vi "gaussian correlation time old.vi"() -> ()   [LabVIEW 2014]
uses:
  <vilib>/userdefined/High Color/IMAQdx.ctl
  <vilib>/Utility/file.llb/Write To Spreadsheet File (DBL).vi
  <vilib>/Utility/file.llb/Read From Spreadsheet File (string).vi
  <vilib>/vision/driver/NI_Vision_Acquisition_Software.lvlib
panel:
  in  "Transfer and Run Date Folder After Experiment":bool
  in  "SSH user name":string
  in  "SSH password":string
  in  "Tags":string
  in  "Wait before recording (s)":dbl
  in  "Correlation Time (s)":dbl
  in  "Start Recording":bool
  in  "Max Power (uW/mm^2)":dbl
  in  "Min Power (uW/mm^2)":dbl
  in  "Frames":i32
  in  "Sigma (uW/mm^2)":dbl
  in  "Offset Power (uW/mm^2)":dbl
  out "Error":string
  out "Save Directory":path
  out "Buffer Number Out":u32
  out "Image":T1(plugin-control)
  in  "stop":bool
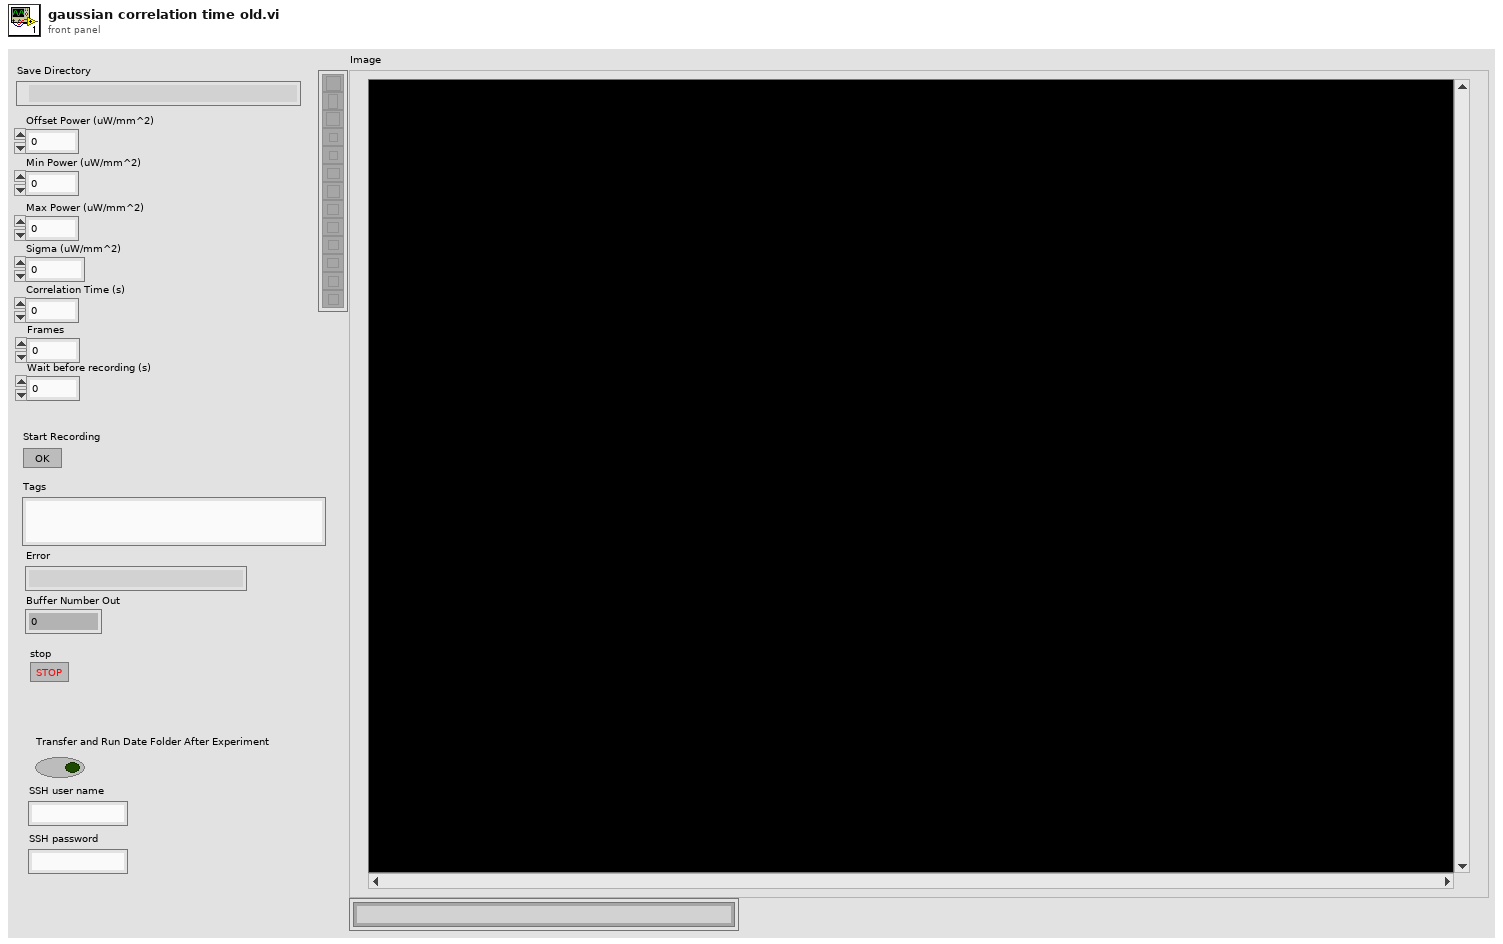
[diagram p1: front panel]
types:
  T1 = typedef "IMAQ Image.ctl" = refnum<image>
  T2 = typedef "IMAQdx.ctl" = refnum<k21>
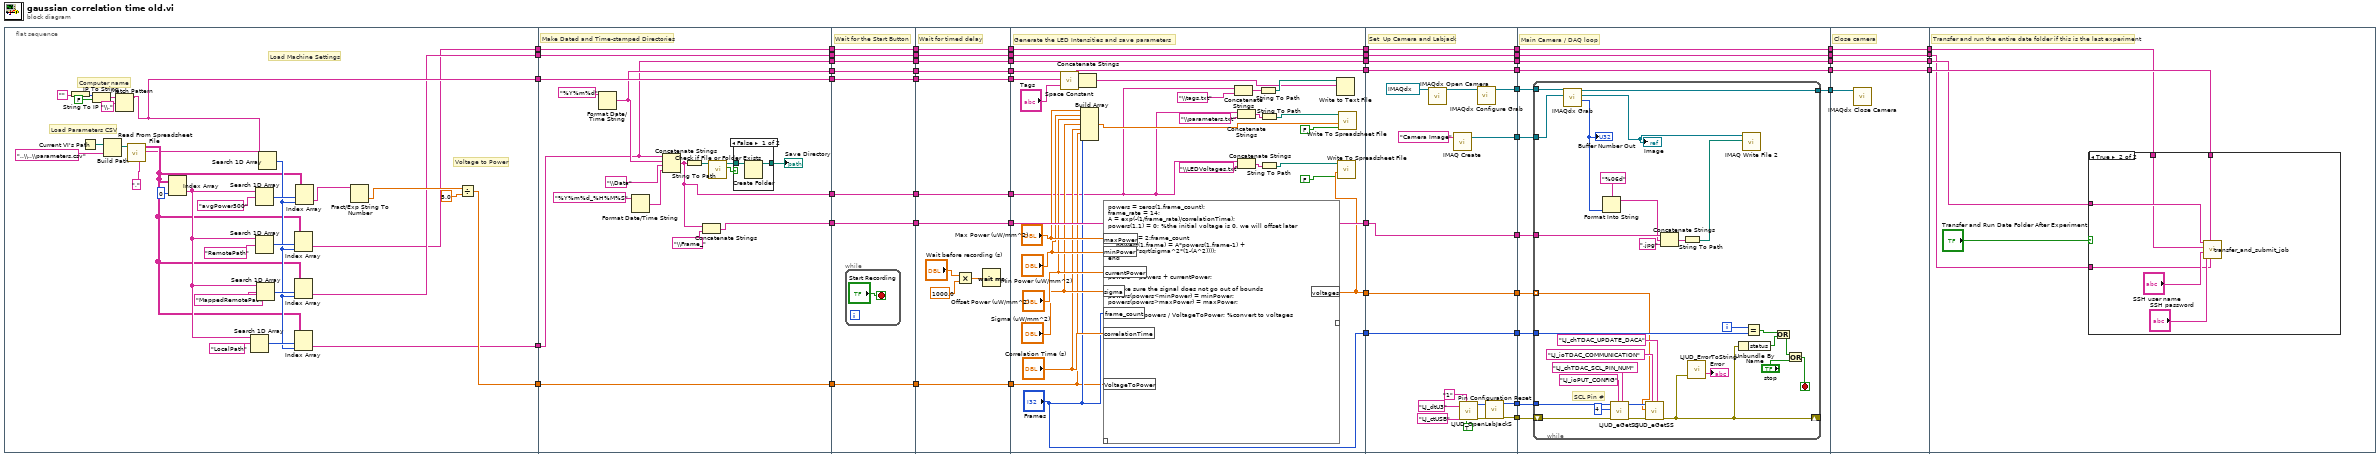
[diagram p0: block diagram]
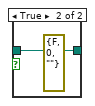
[diagram p2: hidden frame]
diagram:
  n1 = flat-sequence {
    tunnel: [w78] -> w36
    tunnel: [w77] -> w32
    tunnel: [w64] -> w17
    tunnel: [w63] -> w16
    tunnel: [w62] -> w15
    tunnel: [w95] -> w45
    tunnel: [w93] -> w44
    tunnel: [w92] -> w37
    tunnel: w36 -> [w92]
    tunnel: [w91] -> w33
    tunnel: w32 -> [w91]
    tunnel: [w90] -> w29
    tunnel: [w89] -> w24
    tunnel: w17 -> [w89]
    tunnel: w16 -> [w87]
    tunnel: w15 -> [w88]
    tunnel: [w88] -> w8
    tunnel: [w87] -> w1
    tunnel: w45 -> [w114]
    tunnel: [w114] -> w43
    tunnel: w44 -> [w113]
    tunnel: [w113] -> w41
    tunnel: [w112] -> w38
    tunnel: w37 -> [w112]
    tunnel: [w111] -> w34
    tunnel: w33 -> [w111]
    tunnel: [w110] -> w30
    tunnel: w29 -> [w110]
    tunnel: w24 -> [w109]
    tunnel: [w109] -> w18
    tunnel: [w108] -> w9
    tunnel: w8 -> [w108]
    tunnel: [w107] -> w2
    tunnel: w1 -> [w107]
    tunnel: w43 -> [w126]
    tunnel: [w126] -> w42
    tunnel: w41 -> [w125]
    tunnel: [w125] -> w40
    tunnel: [w121] -> w39
    tunnel: w38 -> [w121]
    tunnel: [w120] -> w35
    tunnel: w34 -> [w120]
    tunnel: [w119] -> w31
    tunnel: w30 -> [w119]
    tunnel: [w118] -> w19
    tunnel: w18 -> [w118]
    tunnel: [w117] -> w10
    tunnel: w9 -> [w117]
    tunnel: [w116] -> w3
    tunnel: w2 -> [w116]
    tunnel: w42 -> [w154]
    tunnel: [w154] -> w50
    tunnel: [w152] -> w48
    tunnel: ["Frames"] -> w47
    tunnel: w40 -> [w138]
    tunnel: w39 -> [w139]
    tunnel: w35 -> [w134]
    tunnel: w31 -> [w130]
    tunnel: [w130] -> w25
    tunnel: [w129] -> w20
    tunnel: w19 -> [w129]
    tunnel: [w128] -> w11
    tunnel: w10 -> [w128]
    tunnel: [w127] -> w4
    tunnel: w3 -> [w127]
    tunnel: w50 -> [w171]
    tunnel: [w173] -> w56
    tunnel: [w172] -> w55
    tunnel: [w171] -> w54
    tunnel: [w163] -> w52
    tunnel: [w162] -> w51
    tunnel: [w167] -> w49
    tunnel: w48 -> [w167]
    tunnel: w47 -> [w166]
    tunnel: [w166] -> w46
    tunnel: [w160] -> w26
    tunnel: w25 -> [w160]
    tunnel: [w159] -> w21
    tunnel: w20 -> [w159]
    tunnel: [w158] -> w12
    tunnel: w11 -> [w158]
    tunnel: [w157] -> w5
    tunnel: w4 -> [w157]
    tunnel: w56 -> [w188]
    tunnel: w55 -> [w187]
    tunnel: w54 -> [w186]
    tunnel: [w185] -> w53
    tunnel: w52 -> [w184]
    tunnel: w51 -> [w183]
    tunnel: w49 -> [w182]
    tunnel: w46 -> [w181]
    tunnel: [w180] -> w27
    tunnel: w26 -> [w180]
    tunnel: [w179] -> w22
    tunnel: w21 -> [w179]
    tunnel: [w178] -> w13
    tunnel: w12 -> [w178]
    tunnel: [w177] -> w6
    tunnel: w5 -> [w177]
    tunnel: w53 -> [w223]
    tunnel: [w222] -> w28
    tunnel: w27 -> [w222]
    tunnel: [w221] -> w23
    tunnel: w22 -> [w221]
    tunnel: [w220] -> w14
    tunnel: w13 -> [w220]
    tunnel: [w219] -> w7
    tunnel: w6 -> [w219]
    tunnel: w28 -> [w227]
    tunnel: w23 -> [w226]
    tunnel: w14 -> [w225]
    tunnel: w7 -> [w224]
    frame #0 {
      # "Voltage to Power"
      # "Load Parameters CSV"
      # "Computer name"
      # "Load Machine Settings"
      n2 = String To IP(1:"") -> (0:w86:u32)
      n3 = Current VI's Path() -> (path=w81:path)
      n4 = IP To String(1:FALSE, 2:w86) -> (0:w83:string)
      n5 = Build Path(base path=w81, name or relative path="..\\..\\parameters.csv") -> (appended path=w60:path)
      n6 = Match Pattern(string=w83, regular expression="\\.") -> (before substring=w77:string)  [unwired: 1 in, 3 out]
      n7 = call-poly <vilib>:"Read From Spreadsheet File.vi"("delimiter (\\t)"=",", "file path (dialog if empty)"=w60) -> ("first row"=w58:string[], "all rows"=w59:string[][])  [unwired: 5 in, 3 out]
      n8 = Index Array(array=w59, index (col)=0) -> (element=w61:string[])  [unwired: 1 in]
      n9 = Search 1D Array(1D array=w61, element="LocalPath") -> (index of element=w66:i32)  [unwired: 1 in]
      n10 = Search 1D Array(1D array=w61, element="RemotePath") -> (index of element=w71:i32)  [unwired: 1 in]
      n11 = Search 1D Array(1D array=w61, element="avgPower500") -> (index of element=w72:i32)  [unwired: 1 in]
      n12 = Search 1D Array(1D array=w61, element="MappedRemotePath") -> (index of element=w70:i32)  [unwired: 1 in]
      n13 = Search 1D Array(1D array=w58, element=w77) -> (index of element=w65:i32)  [unwired: 1 in]
      n14 = Index Array(array=w59, index (row)=w71, index (col)=w65) -> (element=w62:string)
      n15 = Index Array(array=w59, index (row)=w70, index (col)=w65) -> (element=w63:string)
      n16 = Index Array(array=w59, index (row)=w66, index (col)=w65) -> (element=w64:string)
      n17 = Index Array(array=w59, index (row)=w72, index (col)=w65) -> (element=w69:string)
      n18 = Fract/Exp String To Number(string=w69) -> (number=w68:dbl)  [unwired: 3 in, 1 out]
      n19 = Divide(x=w68, y=5.0) -> (x/y=w78:dbl)
    }
    frame #1 {
      # "Make Dated and Time-stamped Directories"
      n20 = Format Date/Time String(time format string (%c)="%Y%m%d") -> (date/time string=w90:string)  [unwired: 2 in]
      n21 = Format Date/Time String(time format string (%c)="%Y%m%d_%H%M%S") -> (date/time string=w98:string)  [unwired: 2 in]
      n22 = Concatenate Strings(w89, w90, "\\Data", w98) -> (w93:string)
      n23 = String To Path(string=w93) -> (path=w97:path)
      n24 = Concatenate Strings(w93, "\\Frame_") -> (w95:string)
      n25 = call <vilib>:"Check if File or Folder Exists.vi"("path"=w97) -> ("file or folder exists?"=w102:bool, "dup path"=w101:path)  [unwired: 8 in, 1 out]
      n26 = case shown="False" w102 {
        tunnel: [w104 w106] -> w96
        tunnel: w101 -> [w105 w106]
        frame False {
          n27 = Create Folder(path (use dialog)=w105) -> (created path=w104:path)  [unwired: 2 in, 2 out]
        }
        frame True {
          (unwired) errorcluster {"status"=FALSE, "code"=0, "source"=""} ("error out")
        }
      }
      "Save Directory" <- w96
    }
    frame #2 {
      # "Wait for the Start Button"
      n28 = while {
        stop <- "Start Recording" stop-if-true
      }
    }
    frame #3 {
      # "Wait for timed delay"
      n29 = Multiply(x="Wait before recording (s)", y=1000.0) -> (x*y=w123:dbl)
      n30 = Wait (ms)(milliseconds to wait=w123) -> ()  [unwired: 1 out]
    }
    frame #4 {
      # "Generate the LED Intensities and save parameters"
      n31 = call <vilib>:"Space Constant.vi"() -> ("String"=w132:string)
      n32 = Concatenate Strings(w134, w132, "Tags") -> (w131:string)
      n33 = Build Array("Max Power (uW/mm^2)", "Min Power (uW/mm^2)", "Offset Power (uW/mm^2)", "Sigma (uW/mm^2)", "Correlation Time (s)", w139, "Frames") -> (w142:dbl[])
      n34 = script code="powers = zeros(1,frame_count);\nframe_rate = 14;\nA = exp(-(1/frame_rate)/correlationTime);\npowers(1,1) = 0; %the initial voltage is 0, we will offset later\n\nfor frame = 2:frame_count\n    powers(1,frame) = A*powers(1,frame-1) + (randn(1)*sqrt(sigma^2*(1-(A^2))));\nend\n\n%offset\npowers = powers + currentPower;\n\n%make sure the signal does not go out of bounds\npowers(powers<minPower) = minPower;\npowers(powers>maxPower) = maxPower;\n\nvoltages = powers / VoltageToPower; %convert to voltages"("currentPower"="Offset Power (uW/mm^2)", "frame_count"="Frames", "sigma"="Sigma (uW/mm^2)", "minPower"="Min Power (uW/mm^2)", "maxPower"="Max Power (uW/mm^2)", "correlationTime"="Correlation Time (s)", "VoltageToPower"=w139) -> ("voltages"=w152:dbl[])  [unwired: 1 in, 1 out]
      n35 = Concatenate Strings(w138, "\\tags.txt") -> (w136:string)
      n36 = Concatenate Strings(w138, "\\LEDVoltages.txt") -> (w156:string)
      n37 = Concatenate Strings(w138, "\\parameters.txt") -> (w146:string)
      n38 = String To Path(string=w136) -> (path=w135:path)
      n39 = String To Path(string=w156) -> (path=w155:path)
      n40 = String To Path(string=w146) -> (path=w145:path)
      n41 = Write to Text File(file (use dialog)=w135, text=w131) -> ()  [unwired: 2 in, 3 out]
      n42 = call-poly <vilib>:"Write To Spreadsheet File.vi"("append to file? (new file:F)"=FALSE, "1D data"=w152, "file path (dialog if empty)"=w155) -> ()  [unwired: 5 in, 1 out]
      n43 = call-poly <vilib>:"Write To Spreadsheet File.vi"("append to file? (new file:F)"=FALSE, "1D data"=w142, "file path (dialog if empty)"=w145) -> ()  [unwired: 5 in, 1 out]
    }
    frame #5 {
      # "Set  Up Camera and Labjack"
      n44 = call <vilib>:"IMAQdx Open Camera.vi"("Session In"=T2 "cam0") -> ("Session Out"=w175:T2)  [unwired: 9 in, 1 out]
      n45 = call "IMAQ Create"("Image Name"="Camera Image") -> ("New Image"=w172:T1)  [unwired: 4 in, 1 out]
      n46 = call "LJUD_OpenLabJackS.vi"("FirstFound"=TRUE, "Address"="1" ("DeviceType"), "ConnectionType"="LJ_ctUSB", "DeviceType"="LJ_dtU3") -> ("error out"=w161:errorcluster, "Handle"=w164:i32)  [unwired: 5 in, 1 out]
      n47 = call <vilib>:"IMAQdx Configure Grab.vi"("Session In"=w175) -> ("Session Out"=w173:T2)  [unwired: 9 in, 1 out]
      n48 = call "Pin Configuration Reset.vi"("error in"=w161, "Handle In"=w164) -> ("error out"=w162:errorcluster, "Handle Out"=w163:i32)  [unwired: 8 in]
    }
    frame #6 {
      # "Main Camera / DAQ loop"
      n49 = while {
        tunnel: w188 -> [w218]
        tunnel: [w217] -> w185
        tunnel: w187 -> [w216]
        tunnel: w186 -> [w214]
        tunnel: w184 -> [w191]
        shift-right: [w192] -> _
        shift-left: w183 -> [w190]
        tunnel: w182 -> [w189] mode=indexing
        tunnel: w181 -> [w200]
        i -> [w201]
        stop <- w207 stop-if-true
        # "SCL Pin #"
        n50 = call <vilib>:"IMAQdx Grab.vi"("Image In"=w216, "Session In"=w218) -> ("Buffer Number Out"=w210:u32, "Image Out"=w215:T1, "Session Out"=w217:T2)  [unwired: 6 in, 1 out]
        "Image" <- w215
        "Buffer Number Out" <- w210
        n51 = Format Into String(format string="%06d" ("string"), w210) -> (resulting string=w209:string)  [unwired: 2 in, 1 out]
        n52 = call "LJUD_eGetSS.vi"("Channel"="LJ_chTDAC_SCL_PIN_NUM", "IOType"="LJ_ioPUT_CONFIG", "error in"=w190, "Value Write"=4, "Handle In"=w191) -> ("error out"=w193:errorcluster, "Handle Out"=w196:i32)  [unwired: 4 in, 1 out]
        n53 = call "LJUD_eGetSS.vi"("Channel"="LJ_chTDAC_UPDATE_DACA", "IOType"="LJ_ioTDAC_COMMUNICATION", "error in"=w193, "Value Write"=w189, "Handle In"=w196) -> ("error out"=w192:errorcluster)  [unwired: 4 in, 2 out]
        n54 = Concatenate Strings(w214, w209, ".jpg" ("string")) -> (w212:string)
        n55 = String To Path(string=w212) -> (path=w211:path)
        n56 = call "LJUD_ErrorToString.vi"("error in"=w192) -> ("String"=→"Error":string)  [unwired: 10 in]
        n57 = Unbundle By Name(w192) -> ("status"=w204:bool)
        n58 = call-poly "IMAQ Write File 2"("File Path"=w211, "Image"=w215) -> ()  [unwired: 8 in, 2 out]
        n59 = Equal?(x=w201, y=w200) -> (x = y?=w203:bool)
        n60 = Or(x=w203, y=w204) -> (x .or. y?=w202:bool)
        n61 = Or(x=w202, y="stop") -> (x .or. y?=w207:bool)
      }
    }
    frame #7 {
      # "Close camera"
      n62 = call <vilib>:"IMAQdx Close Camera.vi"("Session In"=w223) -> ()  [unwired: 10 in, 1 out]
    }
    frame #8 {
      # "Transfer and run the entire date folder if this is the last experiment"
      n63 = case shown="True" "Transfer and Run Date Folder After Experiment" {
        tunnel: w227 -> [_ w232]
        tunnel: w226 -> [_ w231]
        tunnel: w225 -> [_ w230]
        tunnel: w224 -> [_ w229]
        frame False {
        }
        frame True {
          n64 = call "transfer_and_submit_job.vi"("Mapped Remote Directory Path"=w229, "Date Folder"=w232, "Password"="SSH password", "Username"="SSH user name", "Remote Data Directory"=w230, "Local Data Directory"=w231) -> ()  [unwired: 6 in]
        }
      }
    }
  }
